vi "Cal Month Table.vi"(5 "date":cluster{"year":u16, "month":u16}) -> (2 "month table":cluster{"selected":bool, "day":string}[][](array[cluster]))   [LabVIEW 2020]
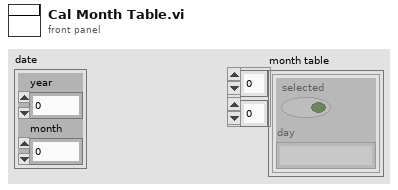
[diagram p1: front panel]
types:
  T1 = cluster{"year":u16, "month":u16, "day of month":u16}
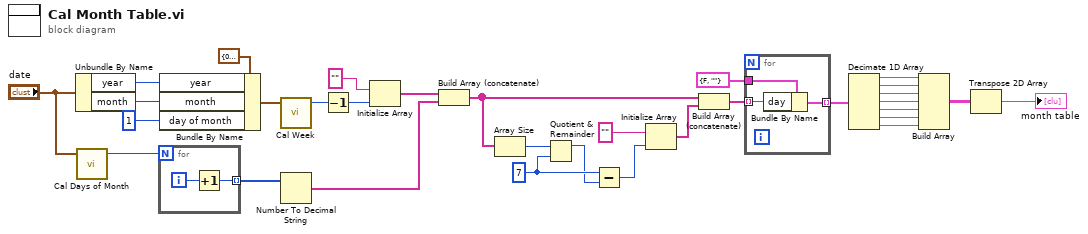
[diagram p0: block diagram]
diagram:
  w8 = 7 ("y")
  n1 = Unbundle By Name("date") -> ("year"=w28:u16, "month"=w29:u16)
  n2 = call "Cal Days of Month.vi"("date"="date") -> ("days"=w23:u16)  [unwired: 4 in]
  n3 = for {
    N: w23 -> [_]
    tunnel: [w33] -> w22 mode=indexing
    i -> [w34]
    n4 = Increment(x=w34) -> (x+1=w33:i32)
  }
  n5 = Bundle By Name(cluster=T1 {"year"=0, "month"=0, "day of month"=0} ("time"), "year"=w28, "month"=w29, "day of month"=u16 1) -> (w30:T1)
  n6 = call "Cal Week.vi"("time"=w30) -> ("week"=w26:u16)  [unwired: 4 in]
  n7 = Number To Decimal String(number=w22) -> (decimal integer string=w12:string[])  [unwired: 1 in]
  n8 = Decrement(x=w26) -> (x-1=w25:u16)
  n9 = Initialize Array("", w25) -> (w13:string[])
  n10 = Build Array (concatenate)(w13, w12) -> (w10:string[])
  n11 = Array Size(array=w10) -> (size(s)=w11:i32)
  n12 = Quotient & Remainder(x=w11, y=w8) -> (x-y*floor(x/y)=w7:i32)  [unwired: 1 out]
  n13 = Subtract(x=w8, y=w7) -> (x-y=w6:i32)
  n14 = Initialize Array("" ("element"), w6) -> (w9:string[])
  n15 = Build Array (concatenate)(w10, w9) -> (w4:string[])
  n16 = for {
    tunnel: w4 -> [w36] mode=indexing
    tunnel: cluster{"selected":bool, "day":string} {"selected"=FALSE, "day"=""} -> [w37]
    tunnel: [w35] -> w3 mode=indexing
    n17 = Bundle By Name(cluster=w37, "day"=w36) -> (w35:cluster{"selected":bool, "day":string})
  }
  n18 = Decimate 1D Array(w3) -> (w21:cluster{"selected":bool, "day":string}[], w20:cluster{"selected":bool, "day":string}[], w19:cluster{"selected":bool, "day":string}[], w18:cluster{"selected":bool, "day":string}[], w17:cluster{"selected":bool, "day":string}[], w16:cluster{"selected":bool, "day":string}[], w15:cluster{"selected":bool, "day":string}[])
  n19 = Build Array(w21, w20, w19, w18, w17, w16, w15) -> (w14:cluster{"selected":bool, "day":string}[][])
  n20 = Transpose 2D Array(2D array=w14) -> (transposed array=→"month table":cluster{"selected":bool, "day":string}[][])
